vi "Main.vi"() -> ()   [LabVIEW 2015]
uses:
  <vilib>/vision/Measure.llb/Edge New.ctl
  <vilib>/vision/Measure.llb/Edge Options.ctl
  <vilib>/vision/Measure.llb/Edge Polarity.ctl
  <vilib>/vision/NI_Vision_Development_Module.lvlib
panel:
  out "Ekscentryczność":dbl
  out "Przesunięcie [um]":dbl
  out "Kołowość":dbl
  out "Major axis":dbl
  out "Minor axis":dbl
  in  "Field of view":dbl
  in  "STOP":bool
  in  "START":bool
  in  "File path":path
  out "Array 3":cluster{"Edge Info":T1, "Boolean":bool}[](array[cluster]) {"Edge Info"."Distance (Real-World)" format="%.2f"; "Edge Info"."Location (Real-World)"."Y" format="%.2g"; "Edge Info"."Location (Real-World)"."X" format="%.2f"; "Edge Info"."Noise" format="%.2f"; "Edge Info"."Location (Pixel)"."Y" format="%.2g"; "Edge Info"."Location (Pixel)"."X" format="%.2f"; "Edge Info"."Strength" format="%.2f"; "Edge Info"."Distance (Pixel)" format="%.2f"}
  out "Displayed image":T2(plugin-control)
  out "Points array":cluster{"Edge Info":T1, "Boolean":bool}[](array[cluster]) {"Edge Info"."Distance (Real-World)" format="%.2f"; "Edge Info"."Location (Real-World)"."Y" format="%.2g"; "Edge Info"."Location (Real-World)"."X" format="%.2f"; "Edge Info"."Noise" format="%.2f"; "Edge Info"."Location (Pixel)"."Y" format="%.2g"; "Edge Info"."Location (Pixel)"."X" format="%.2f"; "Edge Info"."Strength" format="%.2f"; "Edge Info"."Distance (Pixel)" format="%.2f"}
  in  "Point nr":i32
  in  "HIDE / SHOW":bool
  out "Original image":T2(plugin-control)
  # "Kliknięcie na zdjęciu spowoduje zaznaczenie \nnajbliższego punktu (widocznego lub ukrytego).\n\nNaciśnięcie przycisku HIDE / SHOW \nlub DOWOLNEGO PRZYCISKU NA KLAWIATURZE \nspowoduje ukrycie / pokazanie zaznaczonego punktu. \n\nDo obliczeń brane są tylko punkty widoczne na zdjęciu."
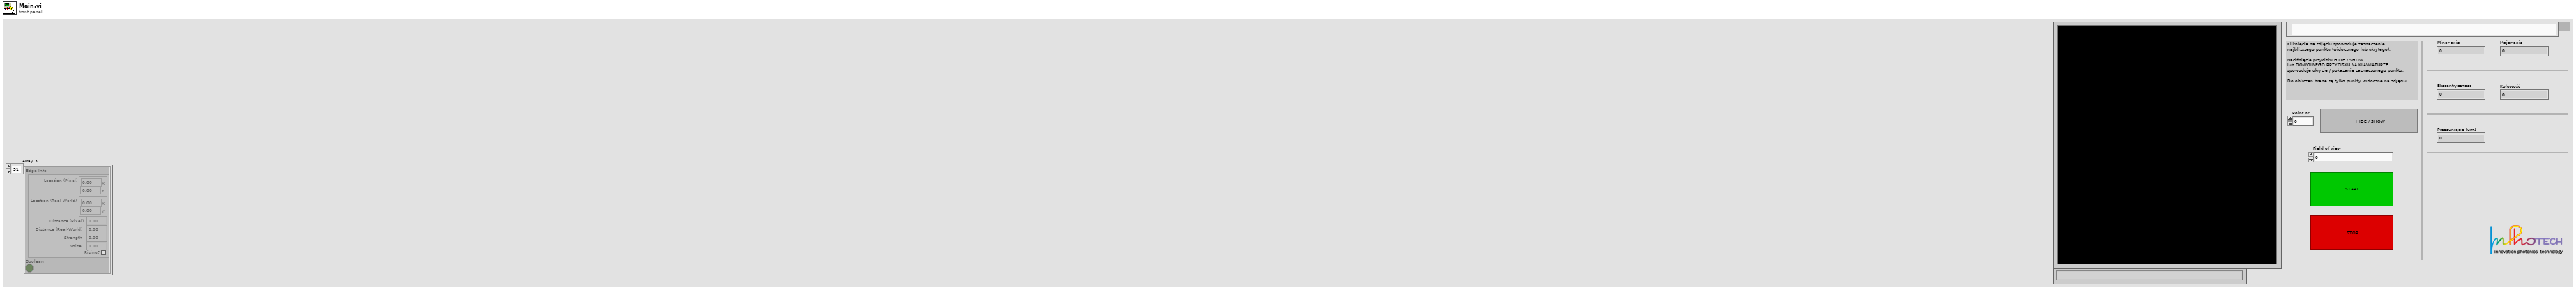
[diagram p1: front panel]
types:
  T1 = typedef "Edge New.ctl" = cluster{"Location (Pixel)":cluster{"X":sgl, "Y":sgl}, "Location (Real-World)":cluster{"X":sgl, "Y":sgl}, "Distance (Pixel)":dbl, "Distance (Real-World)":dbl, "Strength":dbl, "Noise":dbl, "Rising?":bool}
  T2 = typedef "IMAQ Image.ctl" = refnum<image>
  T3 = typedef "Edge Options.ctl" = cluster{"Edge Polarity":T4, "Kernel Size":u32, "Width":u32, "Minimum Edge Strength":sgl, "Interpolation Type":enum32{"Zero Order", "Bilinear", "Quadratic", "Cubic", "Bilinear Fixed"}, "Data Processing Method":enum32{"Average", "Median"}}
  T4 = typedef "Edge Polarity.ctl" = u32
  T5 = cluster{"Search  Direction":u32, "Edge Options":T3, "Show Search Area":bool, "Show Search Lines":bool, "Show Edges Found":bool, "Show Result":bool, "Search Area Color":u32, "Search Lines Color":u32, "Edge Locations Color":u32, "Result Color":u32, "Overlay Group Name":string}
  T6 = typedef "IMAQ Circle" = cluster{"Center X":i32, "Center Y":i32, "Inner Radius":i32, "Outer Radius":i32, "Start Angle":dbl, "End Angle":dbl}
  T7 = typedef "ROI Descriptor" = cluster{"Global Rectangle":i32[], "Contours":cluster{"ID":enum32{"External", "Internal"}, "Type":u32, "Coordinates":i32[]}[]}
  T8 = cluster{"Center":cluster{"X":sgl, "Y":sgl}, "Major Axis":cluster{"Point 1":cluster{"X":sgl, "Y":sgl}, "Point 2":cluster{"X":sgl, "Y":sgl}}, "Minor Axis":cluster{"Point 1":cluster{"X":sgl, "Y":sgl}, "Point 2":cluster{"X":sgl, "Y":sgl}}}
  T9 = cluster{"Center (Pixels)":cluster{"X":sgl, "Y":sgl}, "Radius (Pixels)":dbl, "Center (Real-World)":cluster{"X":sgl, "Y":sgl}, "Radius (Real-World)":dbl, "Roundness (Real-World)":dbl, "Average Strength":dbl, "Average SNR (dB)":dbl}
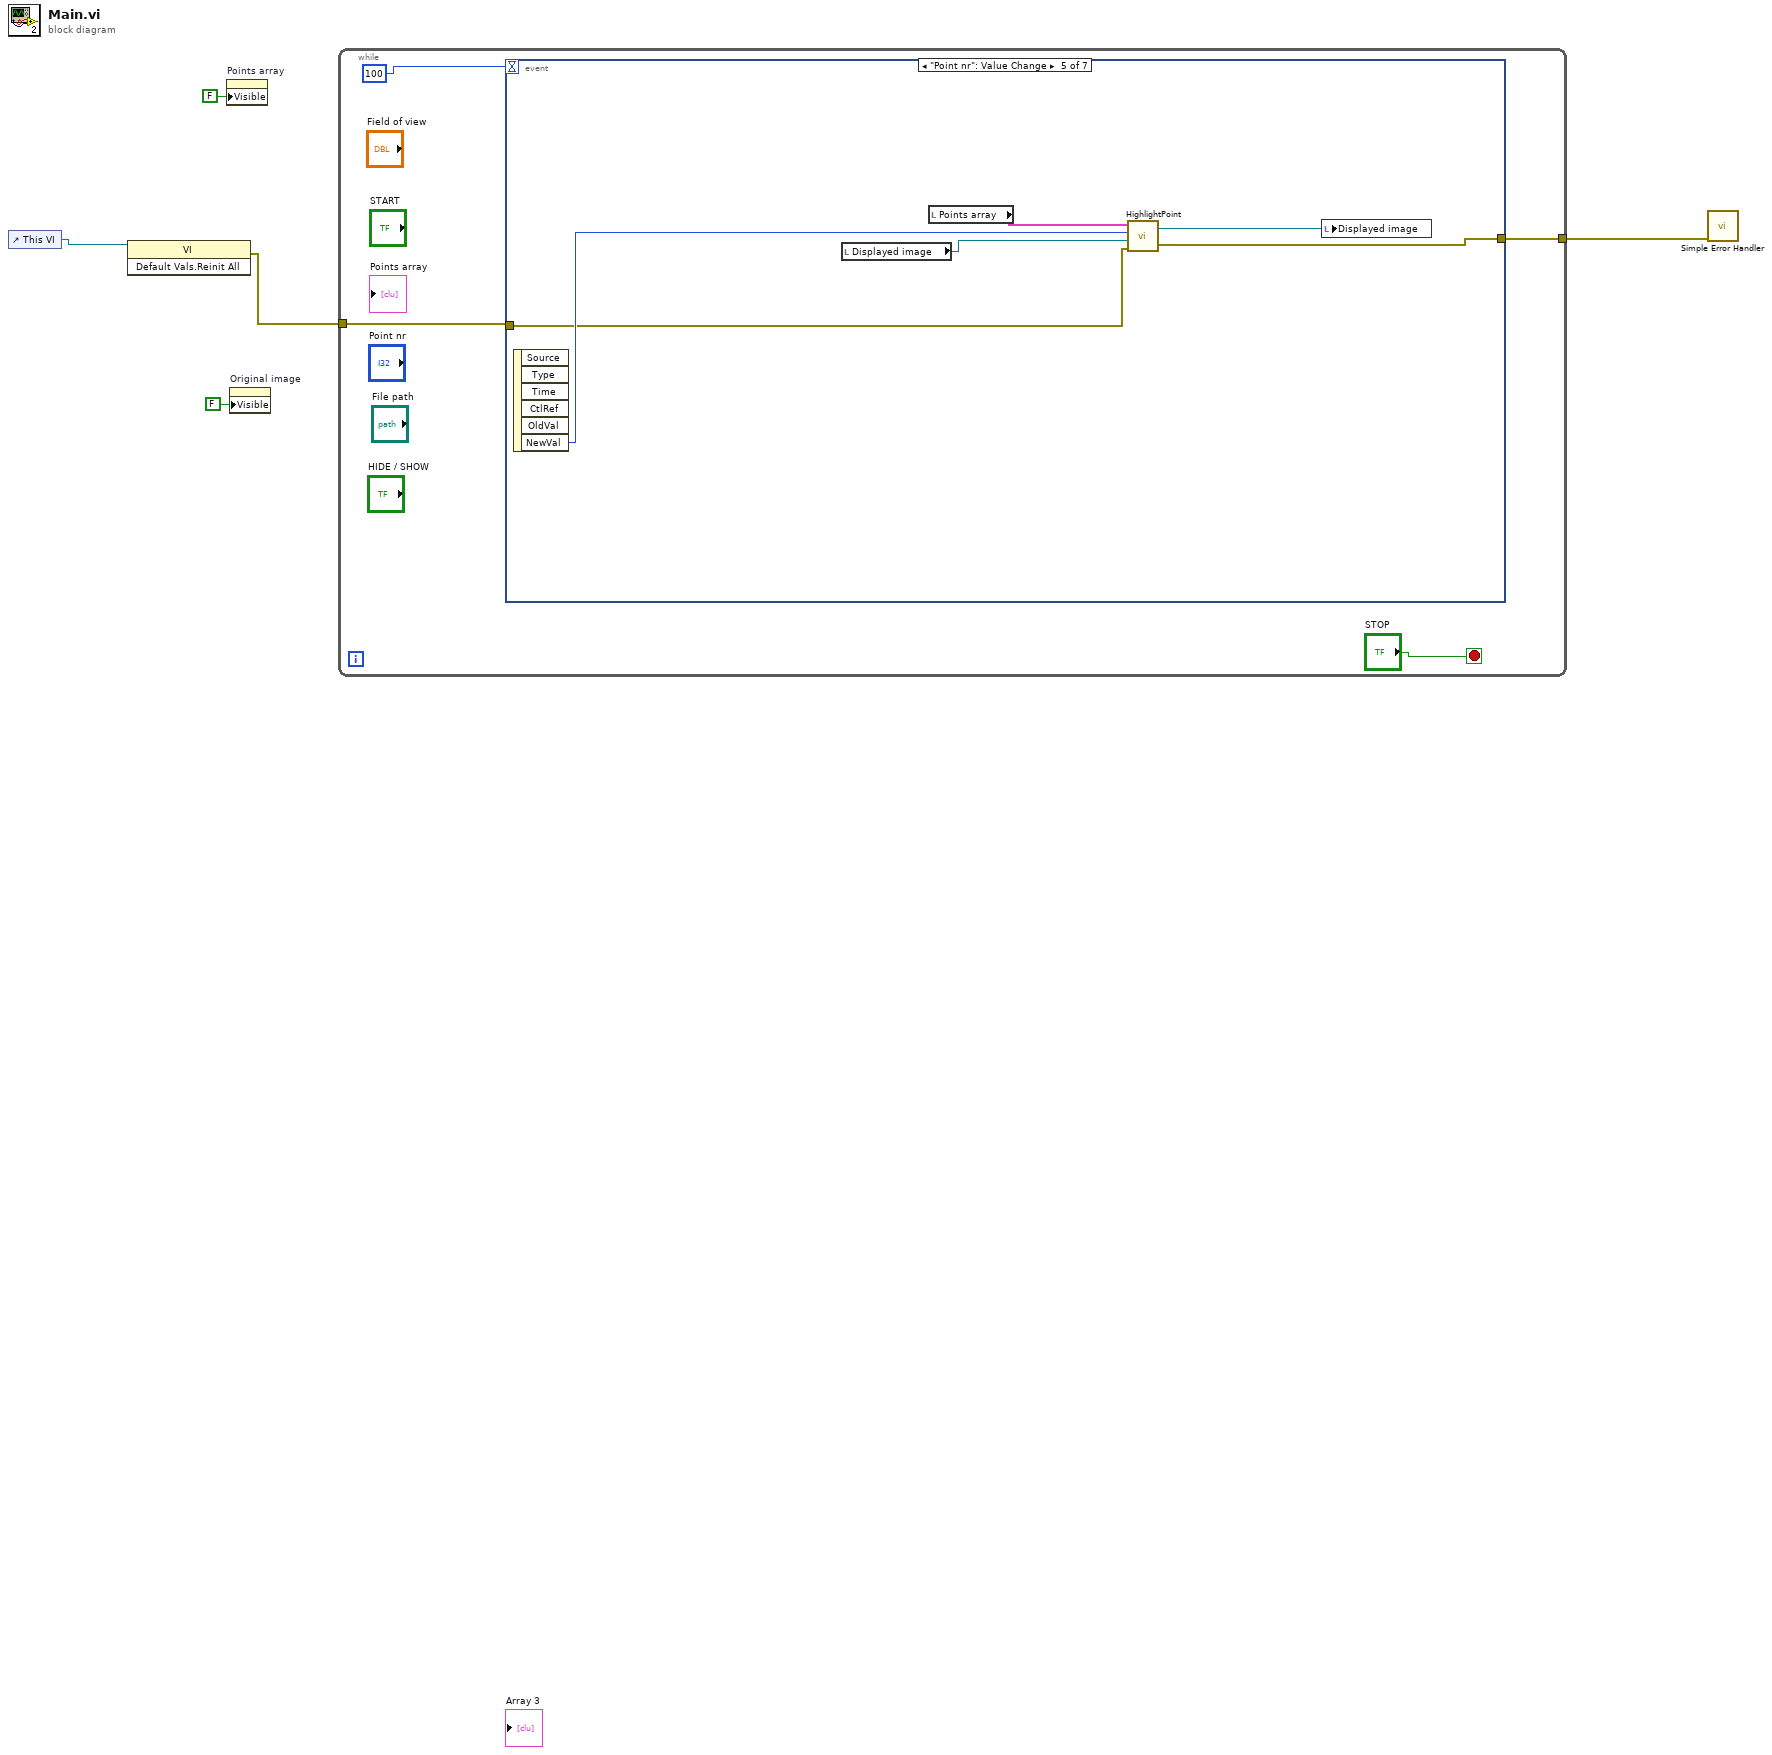
[diagram p0: block diagram]
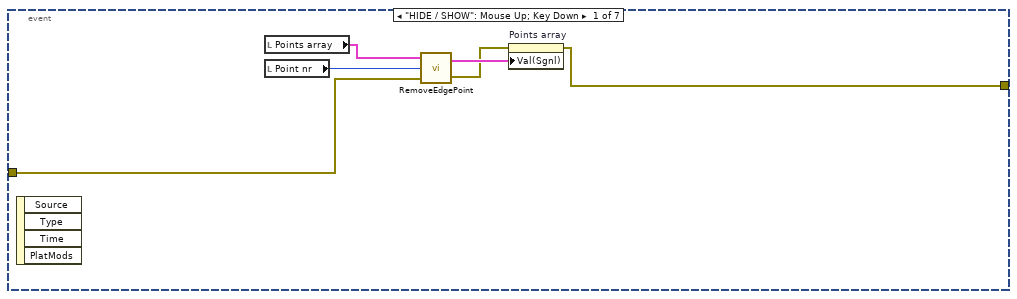
[diagram p2: hidden frame]
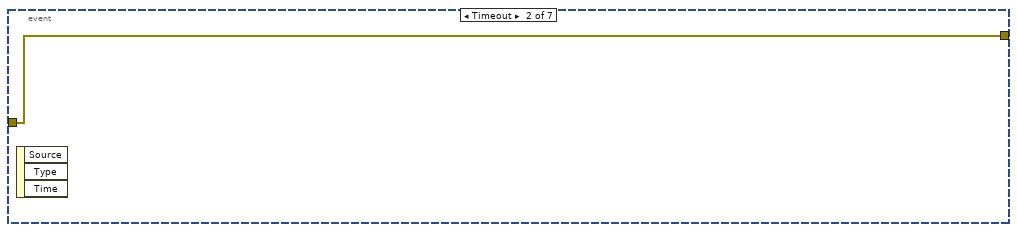
[diagram p3: hidden frame]
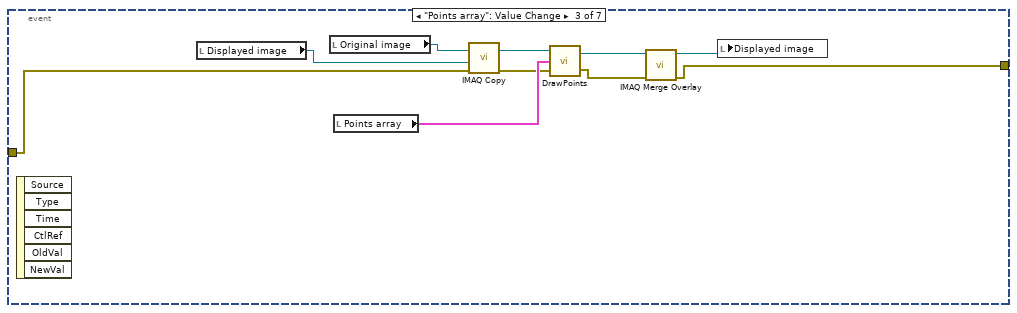
[diagram p4: hidden frame]
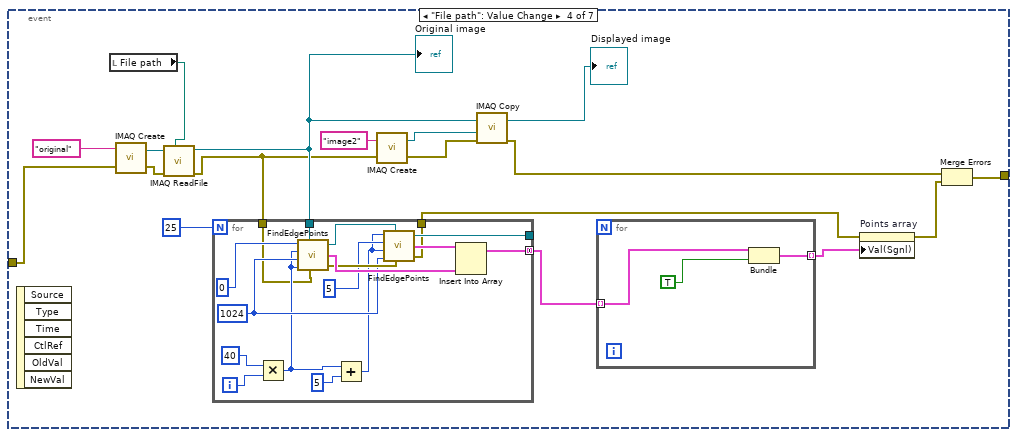
[diagram p5: hidden frame]
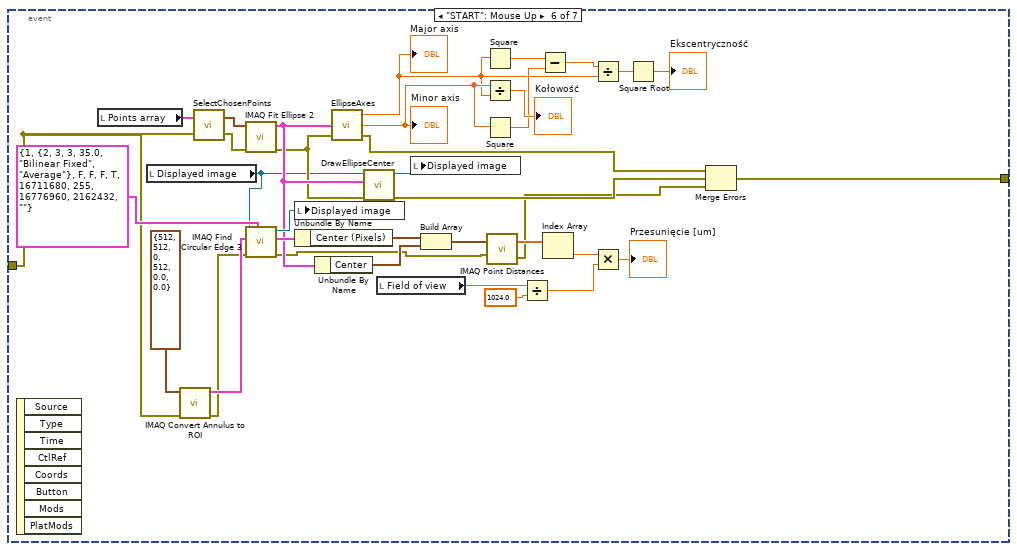
[diagram p6: hidden frame]
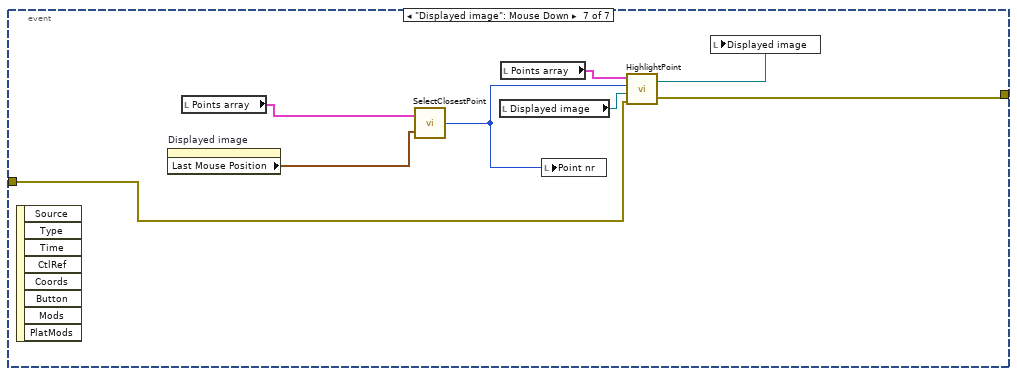
[diagram p7: hidden frame]
diagram:
  n1 = control-ref of="This VI"() -> (w3:refnum<vi>)
  n2 = invoke class="VI" method="Default Vals.Reinit All"(reference=w3) -> (error out=w2:errorcluster)  [unwired: 2 in, 2 out]
  n3 = property on="Points array" class="Arr (strict)"("Visible"=FALSE) -> ()  [unwired: 2 in, 2 out]
  n4 = property on="Original image" class="ImageControl"("Visible"=FALSE) -> ()  [unwired: 2 in, 2 out]
  n5 = while {
    tunnel: w2 -> [w7]
    tunnel: [w6] -> w1
    stop <- "STOP" stop-if-true
    n6 = event shown="[4] \"Point nr\": Value Change" {
      selector: _ -> [_ _ _ _ _ _ _]
      dyn-events: _ -> [_ _ _ _ _ _ _]
      timeout: 100 -> [_ _ _ _ _ _ _]
      tunnel: w7 -> [w10 w16 w20 w34 w66 w79 w107]
      tunnel: [w11 w16 w17 w30 w65 w72 w108] -> w6
      event "HIDE / SHOW": Mouse Up; Key Down {
        n7 = event-data() -> ()  [unwired: 1 in, 4 out]
        n8 = local read "Points array"() -> (w15:cluster{"Edge Info":T1, "Boolean":bool}[])
        n9 = local read "Point nr"() -> (w14:i32)
        n10 = call "RemoveEdgePoint.vi"("error constant"=w10, "index"=w14, "array"=w15) -> ("error constant 2"=w12:errorcluster, "output array"=w13:cluster{"Edge Info":T1, "Boolean":bool}[])
        n11 = property on="Points array" class="Arr (strict)"(error in=w12, "Val(Sgnl)"=w13) -> (error out=w11:errorcluster)  [unwired: 1 in, 1 out]
      }
      event Timeout {
        n12 = event-data() -> ()  [unwired: 1 in, 3 out]
      }
      event "Points array": Value Change {
        n13 = event-data() -> ()  [unwired: 1 in, 6 out]
        n14 = local read "Displayed image"() -> (w25:T2)
        n15 = local read "Original image"() -> (w24:T2)
        n16 = local read "Points array"() -> (w21:cluster{"Edge Info":T1, "Boolean":bool}[])
        n17 = call "IMAQ Copy"("error in (no error)"=w20, "Image Dst"=w25, "Image Src"=w24) -> ("error out"=w19:errorcluster, "Image Dst Out"=w26:T2)  [unwired: 3 in]
        n18 = call "DrawPoints.vi"("error in (no error)"=w19, "Points"=w21, "Image in"=w26) -> ("error out"=w18:errorcluster, "Image Out"=w22:T2)
        n19 = call "IMAQ Merge Overlay"("error in (no error)"=w18, "Image Src"=w22) -> ("error out"=w17:errorcluster, "Image Dst Out"=w23:T2)  [unwired: 8 in]
        n20 = local write "Displayed image"(w23) -> ()
      }
      event "File path": Value Change {
        n21 = event-data() -> ()  [unwired: 1 in, 6 out]
        n22 = local read "File path"() -> (w36:path)
        n23 = call "IMAQ Create"("Image Name"="original", "error in (no error)"=w34) -> ("New Image"=w40:T2, "error out"=w33:errorcluster)  [unwired: 3 in]
        n24 = call "IMAQ ReadFile"("File Path"=w36, "error in (no error)"=w33, "Image"=w40) -> ("error out"=w28:errorcluster, "Image Out"=w44:T2)  [unwired: 4 in, 3 out]
        "Original image" <- w44
        n25 = for {
          N: 25 -> [_]
          tunnel: [w64] -> w37 mode=concatenating
          tunnel: [w59] -> _
          tunnel: w44 -> [w54]
          tunnel: w28 -> [w49]
          tunnel: [w48] -> w27
          i -> [w56]
          w57 = 1024
          n26 = Multiply(x=40, y=w56) -> (x*y=w52:i32)
          n27 = call "FindEdgePoints.vi"("X1"=0, "Image in"=w54, "Y1"=w52, "X2"=w57, "error in (no error)"=w49, "Y2"=w52) -> ("Image out"=w63:T2, "Edge point"=w61:T1[], "error out"=w60:errorcluster)
          n28 = Add(x=w52, y=5) -> (x+y=w50:i32)
          n29 = call "FindEdgePoints.vi"("X1"=w50, "Image in"=w63, "Y1"=5, "X2"=w50, "error in (no error)"=w60, "Y2"=w57) -> ("Image out"=w59:T2, "Edge point"=w62:T1[], "error out"=w48:errorcluster)
          n30 = Insert Into Array(array=w62, new element=w61) -> (w64:T1[])  [unwired: 1 in]
        }
        n31 = call "IMAQ Create"("Image Name"="image2", "error in (no error)"=w28) -> ("New Image"=w43:T2, "error out"=w32:errorcluster)  [unwired: 3 in]
        n32 = call "IMAQ Copy"("error in (no error)"=w32, "Image Dst"=w43, "Image Src"=w44) -> ("error out"=w29:errorcluster, "Image Dst Out"=→"Displayed image":T2)  [unwired: 3 in]
        n33 = for {
          tunnel: w37 -> [w47] mode=indexing
          tunnel: [w46] -> w35 mode=indexing
          n34 = Bundle("Edge Info"=w47, TRUE) -> (w46:cluster{"Edge Info":T1, bool})  [unwired: 1 in]
        }
        n35 = property on="Points array" class="Arr (strict)"(error in=w27, "Val(Sgnl)"=w35) -> (error out=w31:errorcluster)  [unwired: 1 in, 1 out]
        n36 = Merge Errors(w29, w31) -> (w30:errorcluster)
      }
      event "Point nr": Value Change {
        n37 = event-data() -> ("NewVal"=w69:i32)  [unwired: 1 in, 5 out]
        n38 = local read "Displayed image"() -> (w68:T2)
        n39 = local read "Points array"() -> (w70:cluster{"Edge Info":T1, "Boolean":bool}[])
        n40 = call "HighlightPoint.vi"("error in"=w66, "Image In"=w68, "index"=w69, "points"=w70) -> ("error out"=w65:errorcluster, "Image Out"=w67:T2)
        n41 = local write "Displayed image"(w67) -> ()
      }
      event "START": Mouse Up {
        n42 = event-data() -> ()  [unwired: 1 in, 8 out]
        n43 = local read "Points array"() -> (w105:cluster{"Edge Info":T1, "Boolean":bool}[])
        n44 = local read "Displayed image"() -> (w71:T2)
        n45 = call "IMAQ Convert Annulus to ROI"("error in (no error)"=w79, "Annulus"=T6 {"Center X"=512, "Center Y"=512, "Inner Radius"=0, "Outer Radius"=512, "Start Angle"=0.0, "End Angle"=0.0}) -> ("error out"=w78:errorcluster, "ROI Descriptor"=w100:T7)  [unwired: 7 in]
        n46 = call "SelectChosenPoints.vi"("error in (no error)"=w79, "Points array"=w105) -> ("error out"=w80:errorcluster, "array"=w104:cluster{"X":sgl, "Y":sgl}[])
        n47 = call "IMAQ Fit Ellipse 2"("error in (no error)"=w80, "Radial Points"=w104) -> ("error out"=w76:errorcluster, "Ellipse"=w97:T8)  [unwired: 4 in, 4 out]
        n48 = call "IMAQ Find Circular Edge 3"("Options"=T5 {"Search  Direction"=1, "Edge Options"={"Edge Polarity"=2, "Kernel Size"=3, "Width"=3, "Minimum Edge Strength"=35.0, "Interpolation Type"=enum."Bilinear Fixed", "Data Processing Method"=enum."Average"}, "Show Search Area"=FALSE, "Show Search Lines"=FALSE, "Show Edges Found"=FALSE, "Show Result"=TRUE, "Search Area Color"=16711680, "Search Lines Color"=255, "Edge Locations Color"=16776960, "Result Color"=2162432, "Overlay Group Name"=""}, "error in (no error)"=w78, "ROI Descriptor"=w100, "Image"=w71) -> ("error out"=w77:errorcluster, "Fitted Circle"=w98:T9, "Image Out"=w99:T2)  [unwired: 3 in, 2 out]
        n49 = local write "Displayed image"(w99) -> ()
        n50 = Unbundle By Name(w98) -> ("Center (Pixels)"=w96:cluster{"X":sgl, "Y":sgl})
        n51 = Unbundle By Name(w97) -> ("Center"=w95:cluster{"X":sgl, "Y":sgl})
        n52 = call "EllipseAxes.vi"("error in (no error)"=w76, "input cluster"=w97) -> ("error out"=w73:errorcluster, "Minor axis"=w87:dbl, "Major axis"=w83:dbl)  [unwired: 1 in]
        "Minor axis" <- w87
        "Major axis" <- w83
        n53 = call "DrawEllipseCenter.vi"("error in"=w76, "Ellipse"=w97, "Image in"=w71) -> ("error out"=w75:errorcluster, "Image out"=w106:T2)  [unwired: 7 in]
        n54 = local read "Field of view"() -> (w94:dbl)
        n55 = local write "Displayed image"(w106) -> ()
        n56 = Build Array(w96, w95) -> (w92:cluster{"X":sgl, "Y":sgl}[])
        n57 = Square(x=w83) -> (x^2=w86:dbl)
        n58 = Divide(x=w87, y=w83) -> (x/y=→"Kołowość":dbl)
        n59 = Square(x=w87) -> (x^2=w85:dbl)
        n60 = call "IMAQ Point Distances"("Points"=w92, "error in (no error)"=w77) -> ("Distances"=w91:sgl[], "error out"=w74:errorcluster)  [unwired: 3 in]
        n61 = Divide(x=w94, y=1024.0) -> (x/y=w89:dbl)
        n62 = Subtract(x=w86, y=w85) -> (x-y=w84:dbl)
        n63 = Index Array(array=w91) -> (element=w90:sgl)  [unwired: 1 in]
        n64 = Divide(x=w84, y=w83) -> (x/y=w82:dbl)
        n65 = Multiply(x=w90, y=w89) -> (x*y=→"Przesunięcie [um]":dbl)
        n66 = Square Root(x=w82) -> (sqrt(x)=→"Ekscentryczność":dbl)
        n67 = Merge Errors(w73, w75, w74) -> (w72:errorcluster)
      }
      event "Displayed image": Mouse Down {
        n68 = event-data() -> ()  [unwired: 1 in, 8 out]
        n69 = property on="Displayed image" class="ImageControl"() -> ("Last Mouse Position"=w111:cluster{"X":i32, "Y":i32})  [unwired: 2 in, 2 out]
        n70 = local read "Points array"() -> (w110:cluster{"Edge Info":T1, "Boolean":bool}[])
        n71 = call "SelectClosestPoint.vi"("Mouse Position"=w111, "Points"=w110) -> ("Point index"=w109:i32)
        n72 = local read "Displayed image"() -> (w112:T2)
        n73 = local read "Points array"() -> (w114:cluster{"Edge Info":T1, "Boolean":bool}[])
        n74 = local write "Point nr"(w109) -> ()
        n75 = call "HighlightPoint.vi"("error in"=w107, "Image In"=w112, "index"=w109, "points"=w114) -> ("error out"=w108:errorcluster, "Image Out"=w113:T2)
        n76 = local write "Displayed image"(w113) -> ()
      }
    }
  }
  n77 = call <vilib>:"Simple Error Handler.vi"("error in (no error)"=w1) -> ()  [unwired: 4 in, 5 out]
